vi "GCMPlugin_IsSupportingItem.vi"(8 "error in (no error)":errorcluster, 9 "VI Reference":refnum<vi>, 10 "ProjectItem Refnum":refnum<vi>, 11 "_Default in":refnum<class "_EmptyPlugin.lvclass">) -> (0 "error out":errorcluster, 2 "IsSupportingItem":bool, 3 "_Default out":refnum<class "_EmptyPlugin.lvclass">)   [LabVIEW 2014, in "_EmptyPlugin.lvclass"]
uses:
  _EmptyPlugin.lvclass
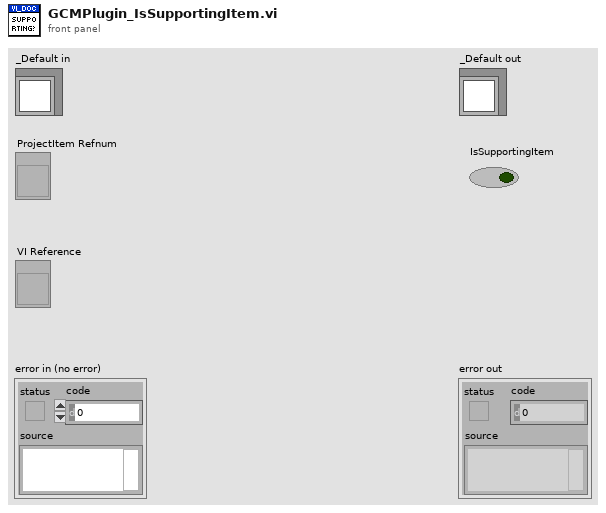
[diagram p1: front panel]
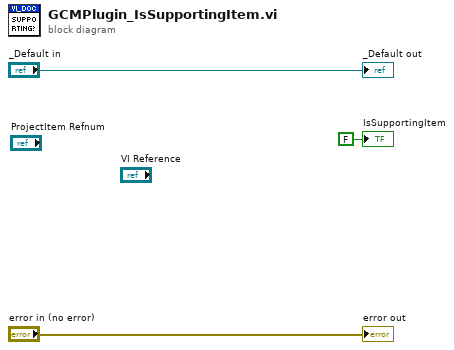
[diagram p0: block diagram]
diagram:
  "error out" <- "error in (no error)"
  "_Default out" <- "_Default in"
  "IsSupportingItem" <- FALSE ("IsSupportingItem")
